vi "Monta comando reentrante .vi"(6 "Set Point":string, 7 "Comando":string, 8 "Dispositivo":string, 9 "Controlador":u16(ring)=1 items=["ZERO", "AH", "DEC", "TUBO", "CUP"]) -> (0 "Erro Comunicação":bool, 1 "String Enviado":string, 2 "Resposta":string, 3 "Erro Resp":bool, 4 "cmdT":string)   [LabVIEW 2018]
uses:
  Global_Telescopio.vi
panel:
  out "ERRO":bool
  # "PROG"
  # "SIDERAL"
  # "EMBREAGEM"
  # "DESLIGAR"
  # "STATUS"
  # "LIGAR"
  # "PARAR"
  # "ERROS"
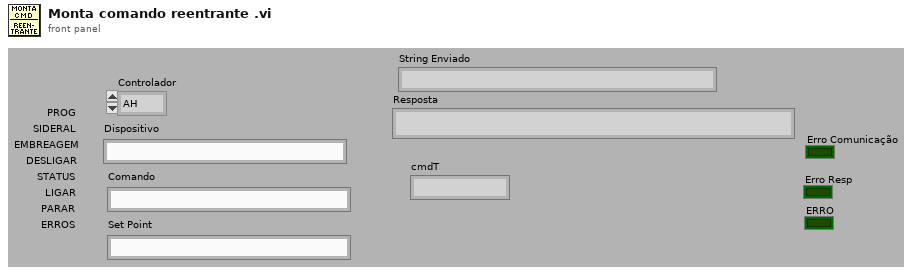
[diagram p1: front panel]
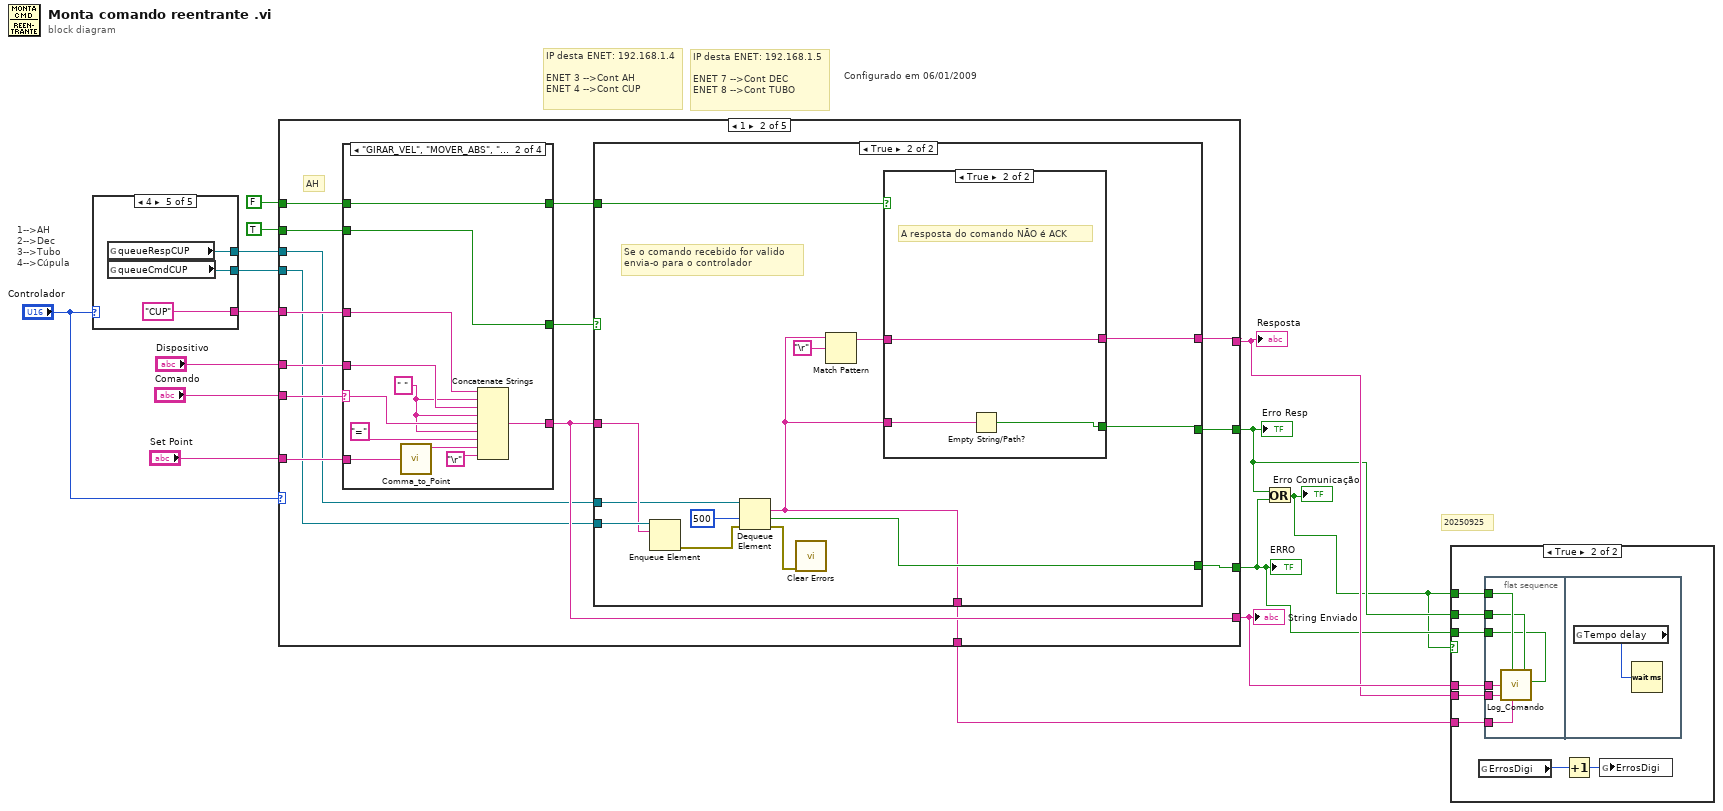
[diagram p0: block diagram]
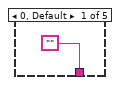
[diagram p3: hidden frame]
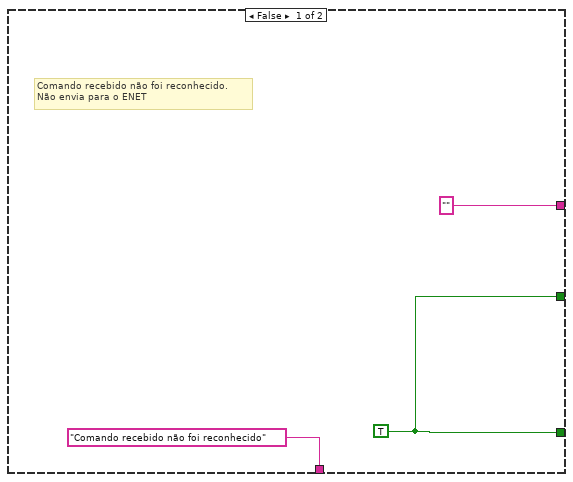
[diagram p4: hidden frame]
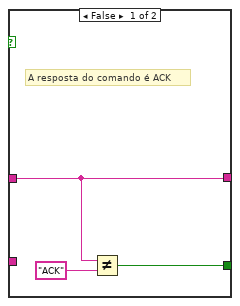
[diagram p5: hidden frame]
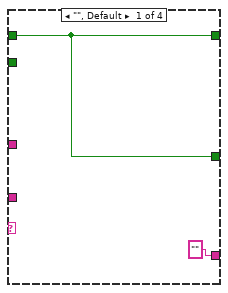
[diagram p6: hidden frame]
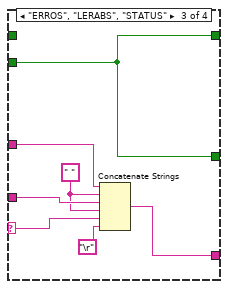
[diagram p7: hidden frame]
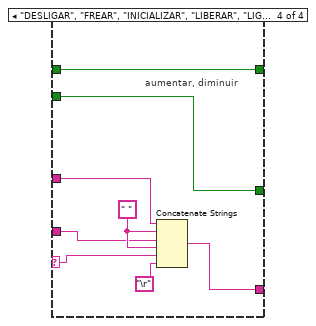
[diagram p8: hidden frame]
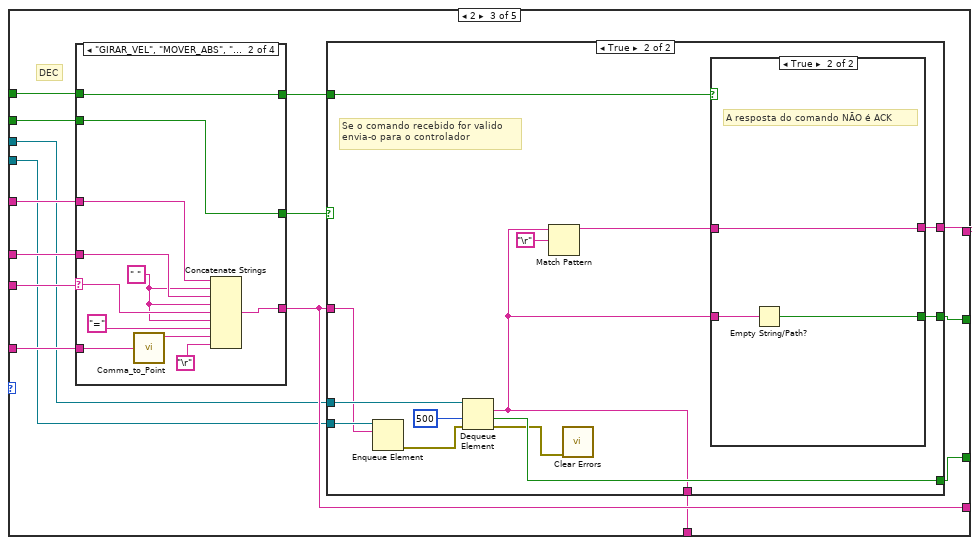
[diagram p9: hidden frame]
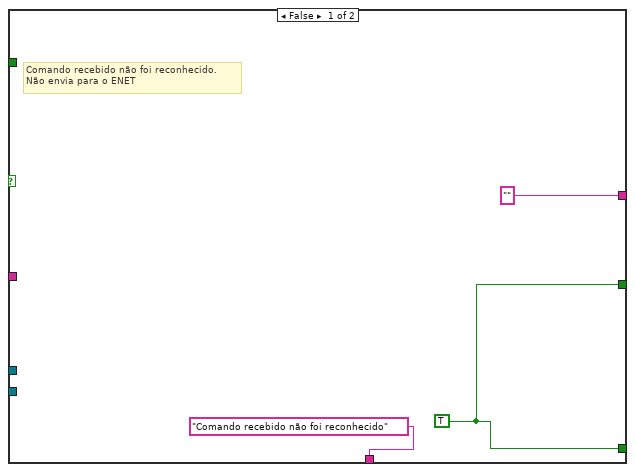
[diagram p10: hidden frame]
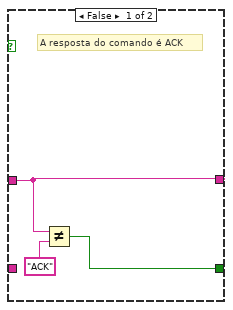
[diagram p11: hidden frame]
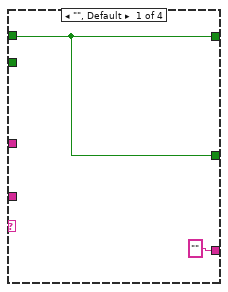
[diagram p12: hidden frame]
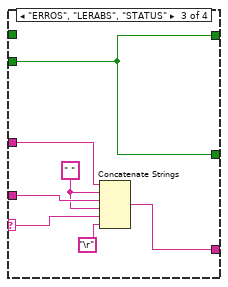
[diagram p13: hidden frame]
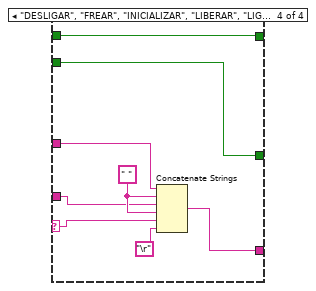
[diagram p14: hidden frame]
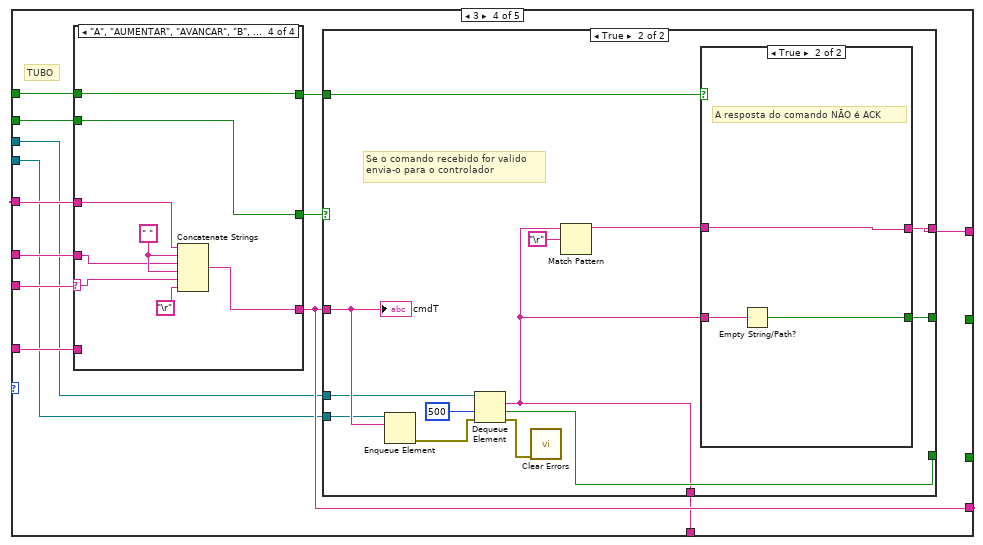
[diagram p15: hidden frame]
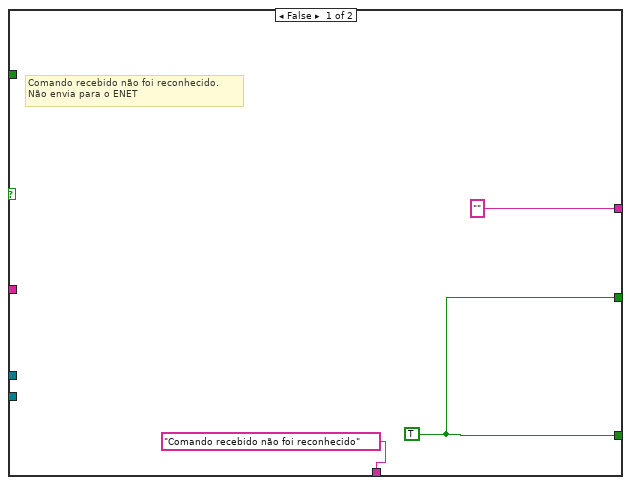
[diagram p16: hidden frame]
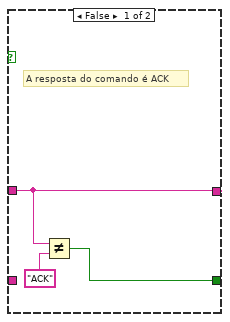
[diagram p17: hidden frame]
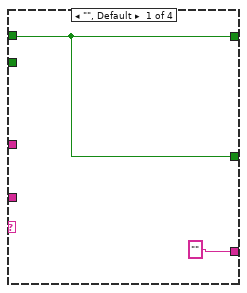
[diagram p18: hidden frame]
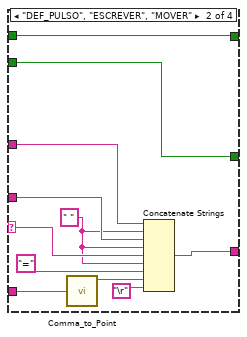
[diagram p19: hidden frame]
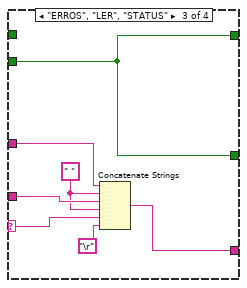
[diagram p20: hidden frame]
diagram:
  # "20250925"
  # "Configurado em 06/01/2009"
  # "IP desta ENET: 192.168.1.4\n\nENET 3 -->Cont AH\nENET 4 -->Cont CUP"
  # "IP desta ENET: 192.168.1.5\n\nENET 7 -->Cont DEC\nENET 8 -->Cont TUBO"
  # "1-->AH\n2-->Dec\n3-->Tubo\n4-->Cúpula"
  n1 = case shown="4" "Controlador" {
    tunnel: ["ZERO" ("string") "AH" ("string") "DEC" ("string") "TUBO" ("string") "CUP" ("string")] -> w11
    tunnel: [_ w18 w21 w24 w26] -> w3
    tunnel: [_ w17 w20 w23 w27] -> w2
    frame 0, Default {
    }
    frame 1 {
      n2 = global read "Global_Telescopio.vi" "queueRespAH"() -> (w17:refnum<queue>)
      n3 = global read "Global_Telescopio.vi" "queueCmdAH"() -> (w18:refnum<queue>)
    }
    frame 2 {
      n4 = global read "Global_Telescopio.vi" "queueCmdDEC"() -> (w21:refnum<queue>)
      n5 = global read "Global_Telescopio.vi" "queueRespDEC"() -> (w20:refnum<queue>)
    }
    frame 3 {
      n6 = global read "Global_Telescopio.vi" "queueRespTUBO"() -> (w23:refnum<queue>)
      n7 = global read "Global_Telescopio.vi" "queueCmdTUBO"() -> (w24:refnum<queue>)
    }
    frame 4 {
      n8 = global read "Global_Telescopio.vi" "queueRespCUP"() -> (w27:refnum<queue>)
      n9 = global read "Global_Telescopio.vi" "queueCmdCUP"() -> (w26:refnum<queue>)
    }
  }
  n10 = case shown="1" "Controlador" {
    tunnel: "Dispositivo" -> [_ w41 w109 w169 w234]
    tunnel: "Comando" -> [_ w40 w107 w168 w233]
    tunnel: "Set Point" -> [_ w39 w108 w167 w232]
    tunnel: w11 -> [_ w42 w106 w170 w235]
    tunnel: [_ w35 w103 w165 w229] -> w7
    tunnel: [_ w37 w101 _ w228] -> w5
    tunnel: [_ w36 w100 _ w230] -> w6
    tunnel: [_ w38 w102 w166 w231] -> w8
    tunnel: FALSE -> [_ w34 w99 w164 w227]
    tunnel: TRUE -> [_ w33 w98 w163 w226]
    tunnel: ["" w32 w97 w162 w225] -> w4
    tunnel: w3 -> [_ w31 w95 w160 w223]
    tunnel: w2 -> [_ w30 w96 w161 w224]
    frame 0, Default {
    }
    frame 1 {
      # "AH"
      n11 = case shown="\"GIRAR_VEL\", \"MOVER_ABS\", \"MOVER_RAP\", \"MOVER_REL\", \"SHIFT\"" w40 {
        selector: w40 -> [_ w76 w83 w89]
        tunnel: w41 -> [_ w79 w84 w90]
        tunnel: w39 -> [_ w78 _ _]
        tunnel: ["" w77 w85 w92] -> w38
        tunnel: w42 -> [_ w75 w81 w91]
        tunnel: [w67 w74 w80 w88] -> w44
        tunnel: w34 -> [w67 w73 _ w87]
        tunnel: w33 -> [_ w74 w80 w88]
        tunnel: [w67 w73 w80 w87] -> w43
        frame "", Default {
        }
        frame "GIRAR_VEL", "MOVER_ABS", "MOVER_RAP", "MOVER_REL", "SHIFT" {
          w72 = " "
          n12 = call "Comma_to_Point.vi"("Lat_A"=w78) -> ("Saída"=w70:string)
          n13 = Concatenate Strings(w75, w72, w79, w72, w76, w72, "=", w70, "\r") -> (w77:string)
        }
        frame "ERROS", "LERABS", "STATUS" {
          w82 = " "
          n14 = Concatenate Strings(w81, w82, w84, w82, w83, "\r") -> (w85:string)
        }
        frame "DESLIGAR", "FREAR", "INICIALIZAR", "LIBERAR", "LIGAR", "PARAR", "RESET", "ZERAR" {
          w93 = " "
          # "aumentar, diminuir"
          n15 = Concatenate Strings(w91, w93, w90, w93, w89, "\r") -> (w92:string)
        }
      }
      n16 = case shown="True" w44 {
        tunnel: ["" w59] -> w35
        tunnel: w38 -> [_ w56]
        tunnel: w43 -> [_ w60]
        tunnel: [w46 w50] -> w37
        tunnel: [w46 w58] -> w36
        tunnel: ["Comando recebido não foi reconhecido" w48] -> w32
        tunnel: w31 -> [_ w57]
        tunnel: w30 -> [_ w53]
        frame False {
          w46 = TRUE
          # "Comando recebido não foi reconhecido.\nNão envia para o ENET"
        }
        frame True {
          # "Se o comando recebido for valido\nenvia-o para o controlador"
          n17 = Enqueue Element(queue=w57, element=w56) -> (error out=w52:errorcluster)  [unwired: 2 in, 2 out]
          n18 = Dequeue Element(queue=w53, timeout in ms (-1)=500, error in (no error)=w52) -> (element=w48:string, timed out?=w50:bool, error out=w49:errorcluster)  [unwired: 1 out]
          n19 = call <vilib>:"Clear Errors.vi"("error in (no error)"=w49) -> ()  [unwired: 5 in, 2 out]
          n20 = Match Pattern(string=w48, regular expression="\r") -> (before substring=w54:string)  [unwired: 1 in, 3 out]
          n21 = case shown="True" w60 {
            tunnel: w54 -> [w62 w66]
            tunnel: [w62 w66] -> w59
            tunnel: [w61 w64] -> w58
            tunnel: w48 -> [_ w65]
            frame False {
              # "A resposta do comando é ACK"
              n22 = Not Equal?(x=w62, y="ACK") -> (x != y?=w61:bool)
            }
            frame True {
              # "A resposta do comando NÃO é ACK"
              n23 = Empty String/Path?(string/path=w65) -> (empty?=w64:bool)
            }
          }
        }
      }
    }
    frame 2 {
      # "DEC"
      n24 = case shown="\"GIRAR_VEL\", \"MOVER_ABS\", \"MOVER_RAP\", \"MOVER_REL\", \"SHIFT\"" w107 {
        selector: w107 -> [_ w141 w148 w154]
        tunnel: w109 -> [_ w144 w149 w155]
        tunnel: w108 -> [_ w143 _ _]
        tunnel: ["" w142 w150 w157] -> w102
        tunnel: w106 -> [_ w140 w146 w156]
        tunnel: [w132 w135 w145 w152] -> w105
        tunnel: w98 -> [_ w135 w145 w152]
        tunnel: w99 -> [w132 w134 _ w153]
        tunnel: [w132 w134 w145 w153] -> w104
        frame "", Default {
        }
        frame "GIRAR_VEL", "MOVER_ABS", "MOVER_RAP", "MOVER_REL", "SHIFT" {
          w139 = " "
          n25 = call "Comma_to_Point.vi"("Lat_A"=w143) -> ("Saída"=w137:string)
          n26 = Concatenate Strings(w140, w139, w144, w139, w141, w139, "=", w137, "\r") -> (w142:string)
        }
        frame "ERROS", "LERABS", "STATUS" {
          w147 = " "
          n27 = Concatenate Strings(w146, w147, w149, w147, w148, "\r") -> (w150:string)
        }
        frame "DESLIGAR", "FREAR", "INICIALIZAR", "LIBERAR", "LIGAR", "PARAR", "RESET", "ZERAR" {
          w158 = " "
          n28 = Concatenate Strings(w156, w158, w155, w158, w154, "\r") -> (w157:string)
        }
      }
      n29 = case shown="True" w105 {
        tunnel: ["" w124] -> w103
        tunnel: w102 -> [_ w115]
        tunnel: w104 -> [_ w125]
        tunnel: [w111 w118] -> w101
        tunnel: [w111 w123] -> w100
        tunnel: ["Comando recebido não foi reconhecido" w113] -> w97
        tunnel: w96 -> [_ w117]
        tunnel: w95 -> [_ w116]
        frame False {
          w111 = TRUE
          # "Comando recebido não foi reconhecido.\nNão envia para o ENET"
        }
        frame True {
          # "Se o comando recebido for valido\nenvia-o para o controlador"
          n30 = Enqueue Element(queue=w116, element=w115) -> (error out=w121:errorcluster)  [unwired: 2 in, 2 out]
          n31 = Dequeue Element(queue=w117, timeout in ms (-1)=500, error in (no error)=w121) -> (element=w113:string, timed out?=w118:bool, error out=w114:errorcluster)  [unwired: 1 out]
          n32 = Match Pattern(string=w113, regular expression="\r") -> (before substring=w119:string)  [unwired: 1 in, 3 out]
          n33 = call <vilib>:"Clear Errors.vi"("error in (no error)"=w114) -> ()  [unwired: 5 in, 2 out]
          n34 = case shown="True" w125 {
            tunnel: w119 -> [w127 w131]
            tunnel: [w127 w131] -> w124
            tunnel: [w126 w130] -> w123
            tunnel: w113 -> [_ w129]
            frame False {
              # "A resposta do comando é ACK"
              n35 = Not Equal?(x=w127, y="ACK") -> (x != y?=w126:bool)
            }
            frame True {
              # "A resposta do comando NÃO é ACK"
              n36 = Empty String/Path?(string/path=w129) -> (empty?=w130:bool)
            }
          }
        }
      }
    }
    frame 3 {
      # "TUBO"
      n37 = case shown="\"A\", \"AUMENTAR\", \"AVANCAR\", \"B\", \"C\", \"DESLIGAR\", \"DIMINUIR\", \"GIRAR\", \"LIGAR\", \"PARAR\", \"RECUAR\", \"RESET\"" w168 {
        selector: w168 -> [_ w204 w211 w217]
        tunnel: w169 -> [_ w207 w212 w218]
        tunnel: w167 -> [_ w206 _ _]
        tunnel: ["" w205 w213 w220] -> w166
        tunnel: w170 -> [_ w203 w209 w219]
        tunnel: [w195 w197 w208 w215] -> w172
        tunnel: w163 -> [_ w197 w208 w215]
        tunnel: w164 -> [w195 w198 _ w216]
        tunnel: [w195 w198 w208 w216] -> w171
        frame "", Default {
        }
        frame "DEF_PULSO", "ESCREVER", "MOVER" {
          w202 = " "
          n38 = call "Comma_to_Point.vi"("Lat_A"=w206) -> ("Saída"=w200:string)
          n39 = Concatenate Strings(w203, w202, w207, w202, w204, w202, "=", w200, "\r") -> (w205:string)
        }
        frame "ERROS", "LER", "STATUS" {
          w210 = " "
          n40 = Concatenate Strings(w209, w210, w212, w210, w211, "\r") -> (w213:string)
        }
        frame "A", "AUMENTAR", "AVANCAR", "B", "C", "DESLIGAR", "DIMINUIR", "GIRAR", "LIGAR", "PARAR", "RECUAR", "RESET" {
          w221 = " "
          n41 = Concatenate Strings(w219, w221, w218, w221, w217, "\r") -> (w220:string)
        }
      }
      n42 = case shown="True" w172 {
        tunnel: ["" w187] -> w165
        tunnel: w166 -> [_ w180]
        tunnel: w171 -> [_ w188]
        tunnel: [w174 w181] -> _
        tunnel: [w174 w186] -> _
        tunnel: ["Comando recebido não foi reconhecido" w176] -> w162
        tunnel: w161 -> [_ w179]
        tunnel: w160 -> [_ w178]
        frame False {
          w174 = TRUE
          # "Comando recebido não foi reconhecido.\nNão envia para o ENET"
        }
        frame True {
          # "Se o comando recebido for valido\nenvia-o para o controlador"
          n43 = Enqueue Element(queue=w178, element=w180) -> (error out=w184:errorcluster)  [unwired: 2 in, 2 out]
          n44 = Dequeue Element(queue=w179, timeout in ms (-1)=500, error in (no error)=w184) -> (element=w176:string, timed out?=w181:bool, error out=w177:errorcluster)  [unwired: 1 out]
          n45 = call <vilib>:"Clear Errors.vi"("error in (no error)"=w177) -> ()  [unwired: 5 in, 2 out]
          n46 = Match Pattern(string=w176, regular expression="\r") -> (before substring=w182:string)  [unwired: 1 in, 3 out]
          n47 = case shown="True" w188 {
            tunnel: w182 -> [w190 w194]
            tunnel: [w190 w194] -> w187
            tunnel: [w189 w193] -> w186
            tunnel: w176 -> [_ w192]
            frame False {
              # "A resposta do comando é ACK"
              n48 = Not Equal?(x=w190, y="ACK") -> (x != y?=w189:bool)
            }
            frame True {
              # "A resposta do comando NÃO é ACK"
              n49 = Empty String/Path?(string/path=w192) -> (empty?=w193:bool)
            }
          }
          "cmdT" <- w180
        }
      }
    }
    frame 4 {
      # "CUP"
      n50 = case shown="\"MOVER\"" w233 {
        selector: w233 -> [_ w269 w276 w282]
        tunnel: w234 -> [_ w272 w277 w283]
        tunnel: w232 -> [_ w271 _ _]
        tunnel: ["" w270 w278 w285] -> w231
        tunnel: w235 -> [_ w268 w274 w284]
        tunnel: [w260 w262 w273 w280] -> w237
        tunnel: w226 -> [_ w262 w273 w280]
        tunnel: w227 -> [w260 w263 _ w281]
        tunnel: [w260 w263 w273 w281] -> w236
        frame "", Default {
        }
        frame "MOVER" {
          w267 = " "
          # "RESP ACK"
          n51 = call "Comma_to_Point.vi"("Lat_A"=w271) -> ("Saída"=w265:string)
          n52 = Concatenate Strings(w268, w267, w272, w267, w269, w267, "=", w265, "\r") -> (w270:string)
        }
        frame "ERROS", "STATUS" {
          w275 = " "
          # "RESP NÃO ACK"
          n53 = Concatenate Strings(w274, w275, w277, w275, w276, "\r") -> (w278:string)
        }
        frame "ABRIR", "DESCER", "DESLIGAR", "FECHAR", "FREAR", "GIRAR_CCW", "GIRAR_CW", "LER_LCB", "LIGAR", "LIGAR_JOG", "LIGAR_LCB", "LIGAR_RAP", "PARAR", "RESET", "SUBIR" {
          w286 = " "
          # "ACK"
          n54 = Concatenate Strings(w284, w286, w283, w286, w282, "\r") -> (w285:string)
        }
      }
      n55 = case shown="True" w237 {
        tunnel: ["" w252] -> w229
        tunnel: w231 -> [_ w245]
        tunnel: w236 -> [_ w253]
        tunnel: [w239 w246] -> w228
        tunnel: [w239 w251] -> w230
        tunnel: ["Comando recebido não foi reconhecido" w241] -> w225
        tunnel: w224 -> [_ w244]
        tunnel: w223 -> [_ w243]
        frame False {
          w239 = TRUE
          # "Comando recebido não foi reconhecido.\nNão envia para o ENET"
        }
        frame True {
          # "Se o comando recebido for valido\nenvia-o para o controlador"
          n56 = Enqueue Element(queue=w243, element=w245) -> (error out=w250:errorcluster)  [unwired: 2 in, 2 out]
          n57 = Dequeue Element(queue=w244, timeout in ms (-1)=500, error in (no error)=w250) -> (element=w241:string, timed out?=w246:bool, error out=w242:errorcluster)  [unwired: 1 out]
          n58 = call <vilib>:"Clear Errors.vi"("error in (no error)"=w242) -> ()  [unwired: 5 in, 2 out]
          n59 = Match Pattern(string=w241, regular expression="\r") -> (before substring=w247:string)  [unwired: 1 in, 3 out]
          n60 = case shown="True" w253 {
            tunnel: w247 -> [w255 w259]
            tunnel: [w255 w259] -> w252
            tunnel: [w254 w258] -> w251
            tunnel: w241 -> [_ w257]
            frame False {
              # "A resposta do comando é ACK"
              n61 = Not Equal?(x=w255, y="ACK") -> (x != y?=w254:bool)
            }
            frame True {
              # "A resposta do comando NÃO é ACK"
              n62 = Empty String/Path?(string/path=w257) -> (empty?=w258:bool)
            }
          }
        }
      }
    }
  }
  "Resposta" <- w7
  "String Enviado" <- w8
  "ERRO" <- w5
  "Erro Resp" <- w6
  n63 = Or(x=w6, y=w5) -> (x .or. y?=w1:bool)
  "Erro Comunicação" <- w1
  n64 = case shown="True" w1 {
    tunnel: w8 -> [_ w295]
    tunnel: w7 -> [_ w294]
    tunnel: w1 -> [_ w293]
    tunnel: w6 -> [_ w292]
    tunnel: w5 -> [_ w291]
    tunnel: w4 -> [_ w290]
    frame False {
    }
    frame True {
      n65 = global read "Global_Telescopio.vi" "ErrosDigi"() -> (w288:i16)
      n66 = flat-sequence {
        tunnel: w295 -> [w301]
        tunnel: w294 -> [w300]
        tunnel: w293 -> [w299]
        tunnel: w292 -> [w298]
        tunnel: w291 -> [w297]
        tunnel: w290 -> [w296]
        frame #0 {
          n67 = call "Log_Comando.vi"("Erro"=w299, "string do Comando"=w301, "string da resposta"=w300, "String"=w296, "Erro de Resposta"=w298, "Erro Recebido"=w297) -> ()  [unwired: 3 in]
        }
        frame #1 {
          n68 = global read "Global_Telescopio.vi" "Tempo delay"() -> (w302:i32)
          n69 = Wait (ms)(milliseconds to wait=w302) -> ()  [unwired: 1 out]
        }
      }
      n70 = Increment(x=w288) -> (x+1=w289:i16)
      n71 = global write "Global_Telescopio.vi" "ErrosDigi"(w289) -> ()
    }
  }
